vi "XY Graph Set Plot Name Event.vi"(8 "Error In":errorcluster, 11 "Plot Name Data":T1) -> (0 "Error Out":errorcluster)   [LabVIEW 2019, in "XY Graph Add-Ons.lvlib"]
uses:
  XY Graph Add-Ons.lvlib
  XY Graph New Plot Name Data.ctl
  XY Graph Refnum.ctl
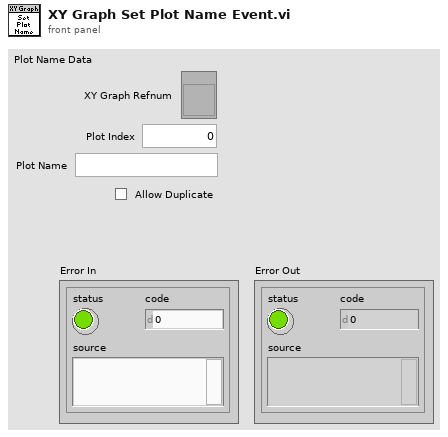
[diagram p1: front panel]
types:
  T1 = typedef "XY Graph Add-Ons.lvlib/XY Graph New Plot Name Data.ctl" = cluster{"XY Graph Refnum":T2, "Plot Index":i32, "Plot Name":string, "Allow Duplicate":bool}
  T2 = typedef "XY Graph Add-Ons.lvlib/XY Graph Refnum.ctl" = refnum<vi>
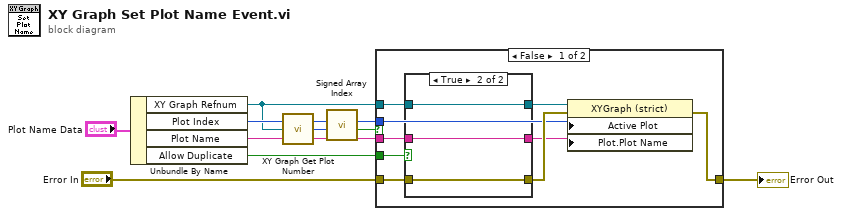
[diagram p0: block diagram]
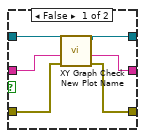
[diagram p2: hidden frame]
diagram:
  n1 = Unbundle By Name("Plot Name Data") -> ("XY Graph Refnum"=w1:T2, "Plot Index"=w9:i32, "Plot Name"=w5:string, "Allow Duplicate"=w4:bool)
  n2 = call "XY Graph Get Plot Number.vi"("XYGraph"=w1) -> ("# Plots"=w8:i32)  [unwired: 8 in]
  n3 = call "Signed Array Index.vi"("Array Size"=w8, "Array Index in"=w9) -> ("Out of Range?"=w7:bool, "Array Index out"=w3:i32)  [unwired: 8 in]
  n4 = case shown="False" w7 {
    tunnel: "Error In" -> [w16 w29]
    tunnel: w5 -> [w17 _]
    tunnel: w4 -> [w18 _]
    tunnel: w3 -> [w13 _]
    tunnel: [w11 w29] -> w2
    tunnel: w1 -> [w19 _]
    frame False {
      n5 = case shown="True" w18 {
        tunnel: w19 -> [w25 w28]
        tunnel: w17 -> [w24 w27]
        tunnel: w16 -> [w23 w26]
        tunnel: [w22 w28] -> w15
        tunnel: [w20 w27] -> w12
        tunnel: [w21 w26] -> w14
        frame False {
          n6 = call "XY Graph Check New Plot Name.vi"("Error In"=w23, "New Plot Name (in)"=w24, "Multiplot XY Graph Refnum in"=w25) -> ("Error Out"=w21:errorcluster, "New Plot Name (out)"=w20:string, "Multiplot XY Graph Refnum out"=w22:refnum<vi>)  [unwired: 6 in]
        }
        frame True {
        }
      }
      n7 = property class="XYGraph (strict)"(reference=w15, error in=w14, "Active Plot"=w13, "Plot.Plot Name"=w12) -> (error out=w11:errorcluster)  [unwired: 1 out]
    }
    frame True {
    }
  }
  "Error Out" <- w2
